vi "method parameters.Facade.vi"(0 "Data In":T5, 2 "Display State In":T3, 3 "Container State":T4) -> (6 "Data Out":T5, 7 "Display State Out":T3, 8 "Action":T2)   [LabVIEW 2014, in "method parameters.xctl"]
uses:
  method parameters.xctl
  method parameters.Data.ctl
  <vilib>/_xctls/Container State.ctl
  method parameters.State.ctl
  <vilib>/_xctls/Action.ctl
  <vilib>/_xctls/XControlSupport.lvlib
  CSlibraries/UtilityLib/UtilityLib.lvlib
  _common/PTUtils/PTUtils.lvlib
  CSCore/CSSystem/CoreLib/CoreLib.lvlib
panel:
  in  "Scrollbar":i32(c297)
  out "Indicator":T1
  in  "Control":T1
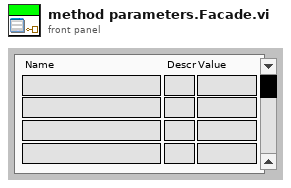
[diagram p1: front panel]
types:
  T1 = cluster{"Name 1":string, "Descr 1":string, "Value 1":string, "Name 2":string, "Descr 2":string, "Value 2":string, "Name 3":string, "Descr 3":string, "Value 3":string, "Name 4":string, "Descr 4":string, "Value 4":string}
  T2 = typedef "XControlSupport.lvlib/Action.ctl" = cluster{"Data Changed?":bool, "State Changed?":bool, "Action Name":string}
  T3 = typedef "method parameters.xctl/method parameters.State.ctl" = cluster{"index":i32}
  T4 = typedef "XControlSupport.lvlib/Container State.ctl" = cluster{"Indicator?":bool, "Run Mode?":bool, " Refnum":refnum<vi>}
  T5 = typedef "method parameters.xctl/method parameters.Data.ctl" = cluster{"Name":string, "Descr":string, "Value":string}[]
  T6 = enum8{"Enabled", "Disabled", "Disabled and Grayed Out"}
  T7 = cluster{"Name":string, "Descr":string, "Value":string}
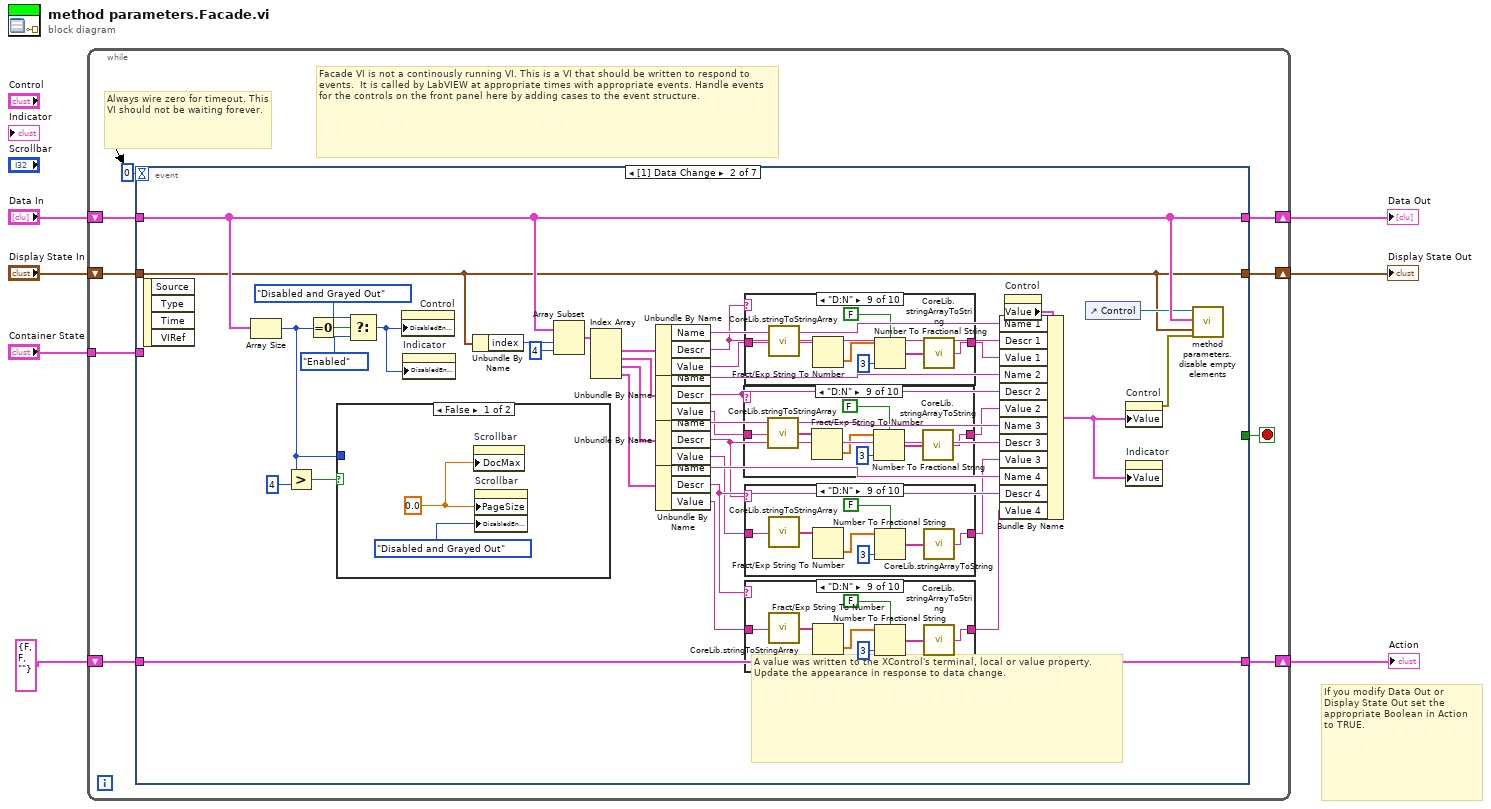
[diagram p0: block diagram]
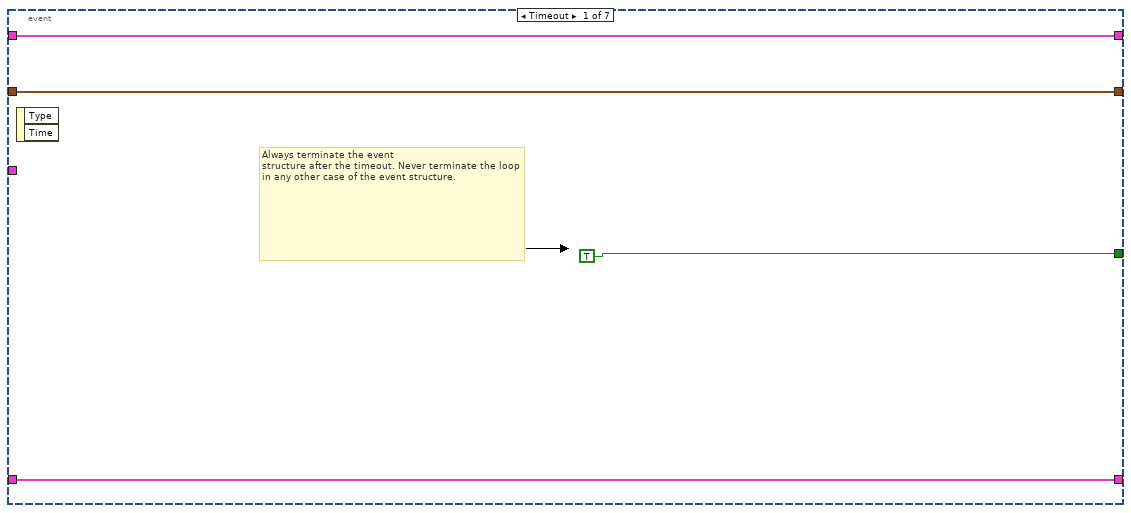
[diagram p2: hidden frame]
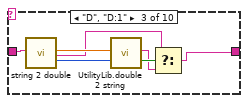
[diagram p5: hidden frame]
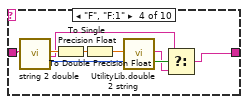
[diagram p6: hidden frame]
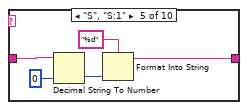
[diagram p7: hidden frame]
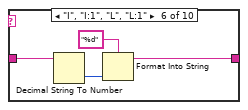
[diagram p8: hidden frame]
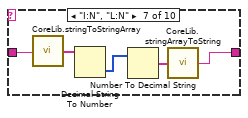
[diagram p9: hidden frame]
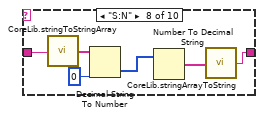
[diagram p10: hidden frame]
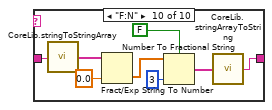
[diagram p11: hidden frame]
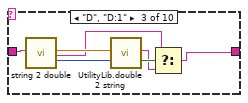
[diagram p14: hidden frame]
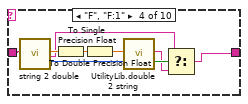
[diagram p15: hidden frame]
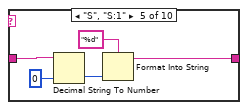
[diagram p16: hidden frame]
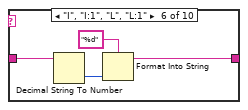
[diagram p17: hidden frame]
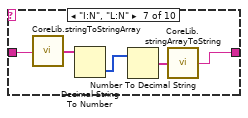
[diagram p18: hidden frame]
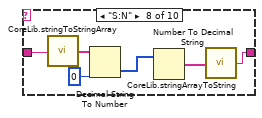
[diagram p19: hidden frame]
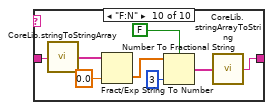
[diagram p20: hidden frame]
diagram:
  # "If you modify Data Out or\nDisplay State Out set the\nappropriate Boolean in Action\nto TRUE."
  n1 = while {
    shift-right: [w15] -> w4
    shift-left: "Display State In" -> [w16]
    tunnel: "Container State" -> [w12]
    shift-right: [w10] -> w7
    shift-left: "Data In" -> [w11]
    shift-right: [w8] -> w2
    shift-left: T2 {"Data Changed?"=FALSE, "State Changed?"=FALSE, "Action Name"=""} ("Action") -> [w9]
    stop <- w14 stop-if-true
    # "Facade VI is not a continously running VI. This is a VI that should be written to respond to events.  It is called by LabVIEW at appropriate times with appropriate events. Handle events for the controls on the front panel here by adding cases to the event structure."
    # "Always wire zero for timeout. This\nVI should not be waiting forever."
    n2 = event shown="[1] Data Change" {
      selector: _ -> [_ _ _ _ _ _ _]
      dyn-events: _ -> [_ _ _ _ _ _ _]
      timeout: 0 -> [_ _ _ _ _ _ _]
      tunnel: w16 -> [w18 w34 w280 w323 w327 w334 w384]
      tunnel: [w18 w34 w280 w323 w327 w329 w384] -> w15
      tunnel: [TRUE _ _ _ _ _ _] -> w14
      tunnel: w12 -> [_ _ _ w324 w328 _ _]
      tunnel: w11 -> [w17 w36 w279 w322 w326 w330 w383]
      tunnel: [w17 w36 w279 w322 w326 w330 w382] -> w10
      tunnel: [w19 w57 w309 w321 w325 w335 w395] -> w8
      tunnel: w9 -> [w19 w57 w309 w321 w325 w336 w396]
      event Timeout {
        # "Always terminate the event\nstructure after the timeout. Never terminate the loop in any other case of the event structure."
        n3 = event-data() -> ()  [unwired: 1 in, 2 out]
      }
      event Data Change {
        # "A value was written to the XControl's terminal, local or value property.\nUpdate the appearance in response to data change."
        n4 = event-data() -> ()  [unwired: 1 in, 4 out]
        n5 = Array Size(array=w36) -> (size(s)=w50:i32)
        n6 = Greater?(x=w50, y=4) -> (0:w56:bool)
        n7 = Equal To 0?(x=w50) -> (x = 0?=w53:bool)
        n8 = case shown="False" w56 {
          tunnel: w50 -> [_ w274]
          frame False {
            w270 = 0.0
            n9 = property on="Scrollbar" class="Scroll (strict)"("DocMax"=w270) -> ()  [unwired: 2 in, 2 out]
            n10 = property on="Scrollbar" class="Scroll (strict)"("PageSize"=w270, "DisabledEnum"=T6."Disabled and Grayed Out" ("Disabled")) -> ()  [unwired: 2 in, 2 out]
          }
          frame True {
            n11 = Subtract(x=w274, y=3) -> (x-y=w276:i32)
            n12 = To Double Precision Float(number=w274) -> (double precision float=w273:dbl)
            n13 = To Double Precision Float(number=w276) -> (double precision float=w275:dbl)
            n14 = property on="Scrollbar" class="Scroll (strict)"("DocMax"=w275, "DisabledEnum"=T6."Enabled" ("Disabled")) -> ()  [unwired: 2 in, 2 out]
            n15 = Divide(x=w275, y=w273) -> (x/y=w277:dbl)
            n16 = property on="Scrollbar" class="Scroll (strict)"("PageSize"=w277) -> ()  [unwired: 2 in, 2 out]
          }
        }
        n17 = Select(t=T6."Disabled and Grayed Out" ("Disabled"), s=w53, f=T6."Enabled" ("Disabled")) -> (s? t:f=w54:T6)
        n18 = property on="Control" class="Clust (strict)"("DisabledEnum"=w54) -> ()  [unwired: 2 in, 2 out]
        n19 = property on="Indicator" class="Clust (strict)"("DisabledEnum"=w54) -> ()  [unwired: 2 in, 2 out]
        n20 = Unbundle By Name(w34) -> ("index"=w48:i32)
        n21 = Array Subset(array=w36, index=w48, length=4) -> (w43:T5)
        n22 = Index Array(array=w43) -> (element #1=w42:T7, element #2=w41:T7, element #3=w40:T7, element #4=w39:T7)  [unwired: 4 in]
        n23 = Unbundle By Name(w42) -> ("Name"=w44:string, "Descr"=w32:string, "Value"=w31:string)
        n24 = Unbundle By Name(w41) -> ("Name"=w45:string, "Descr"=w21:string, "Value"=w23:string)
        n25 = Unbundle By Name(w40) -> ("Name"=w46:string, "Descr"=w25:string, "Value"=w26:string)
        n26 = Unbundle By Name(w39) -> ("Name"=w47:string, "Descr"=w27:string, "Value"=w29:string)
        n27 = case shown="\"D:N\"" w21 {
          tunnel: [w164 w165 w166 w173 w183 w188 w192 w200 w208 w216] -> w22
          tunnel: w23 -> [w164 w165 w170 w177 w182 w187 w191 w196 w203 w210]
          frame Default {
          }
          frame "C", "C:1", "C:N" {
          }
          frame "D", "D:1" {
            n28 = call "string 2 double.vi"("string"=w170) -> ("number"=w171:dbl, "scanned string"=w167:string, "length"=w172:u8)  [unwired: 15 in, 1 out]
            n29 = call "UtilityLib.double 2 string.vi"("Numeric"=w171, "length"=w172) -> ("String"=w168:string, "loss free"=w169:bool)  [unwired: 16 in]
            n30 = Select(t=w167, s=w169, f=w168) -> (s? t:f=w166:string)
          }
          frame "F", "F:1" {
            n31 = call "string 2 double.vi"("string"=w177) -> ("number"=w179:dbl, "scanned string"=w174:string, "length"=w181:u8)  [unwired: 15 in, 1 out]
            n32 = To Single Precision Float(number=w179) -> (single precision float=w180:sgl)
            n33 = To Double Precision Float(number=w180) -> (double precision float=w178:dbl)
            n34 = call "UtilityLib.double 2 string.vi"("Numeric"=w178, "length"=w181) -> ("String"=w175:string, "loss free"=w176:bool)  [unwired: 16 in]
            n35 = Select(t=w174, s=w176, f=w175) -> (s? t:f=w173:string)
          }
          frame "S", "S:1" {
            n36 = Decimal String To Number(string=w182, default (0L)=i16 0) -> (number=w185:i16)  [unwired: 1 in, 1 out]
            n37 = Format Into String(format string="%d", w185) -> (resulting string=w183:string)  [unwired: 2 in, 1 out]
          }
          frame "I", "I:1", "L", "L:1" {
            n38 = Decimal String To Number(string=w187) -> (number=w190:i32)  [unwired: 2 in, 1 out]
            n39 = Format Into String(format string="%d", w190) -> (resulting string=w188:string)  [unwired: 2 in, 1 out]
          }
          frame "I:N", "L:N" {
            n40 = call "CoreLib.stringToStringArray.vi"("String"=w191) -> ("Array"=w195:string[])
            n41 = Decimal String To Number(string=w195) -> (number=w194:i32[])  [unwired: 2 in, 1 out]
            n42 = Number To Decimal String(number=w194) -> (decimal integer string=w193:string[])  [unwired: 1 in]
            n43 = call "CoreLib.stringArrayToString.vi"("Array"=w193) -> ("String"=w192:string)
          }
          frame "S:N" {
            n44 = call "CoreLib.stringToStringArray.vi"("String"=w196) -> ("Array"=w201:string[])
            n45 = Decimal String To Number(string=w201, default (0L)=i16 0 ("default (0 I32)")) -> (number=w198:i16[])  [unwired: 1 in, 1 out]
            n46 = Number To Decimal String(number=w198) -> (decimal integer string=w197:string[])  [unwired: 1 in]
            n47 = call "CoreLib.stringArrayToString.vi"("Array"=w197) -> ("String"=w200:string)
          }
          frame "D:N" {
            n48 = call "CoreLib.stringToStringArray.vi"("String"=w203) -> ("Array"=w206:string[])
            n49 = Fract/Exp String To Number(string=w206) -> (number=w205:dbl[])  [unwired: 3 in, 1 out]
            n50 = Number To Fractional String(use system decimal point (T)=FALSE, number=w205, precision (6)=i16 3) -> (F-format string=w204:string[])  [unwired: 1 in]
            n51 = call "CoreLib.stringArrayToString.vi"("Array"=w204) -> ("String"=w208:string)
          }
          frame "F:N" {
            n52 = call "CoreLib.stringToStringArray.vi"("String"=w210) -> ("Array"=w214:string[])
            n53 = Fract/Exp String To Number(string=w214, default (0 dbl)=sgl 0.0 ("default (0 DBL)")) -> (number=w211:sgl[])  [unwired: 2 in, 1 out]
            n54 = Number To Fractional String(use system decimal point (T)=FALSE, number=w211, precision (6)=i16 3) -> (F-format string=w213:string[])  [unwired: 1 in]
            n55 = call "CoreLib.stringArrayToString.vi"("Array"=w213) -> ("String"=w216:string)
          }
        }
        n56 = case shown="\"D:N\"" w32 {
          tunnel: [w217 w218 w219 w226 w236 w241 w245 w253 w261 w269] -> w30
          tunnel: w31 -> [w217 w218 w223 w230 w235 w240 w244 w249 w256 w263]
          frame Default {
          }
          frame "C", "C:1", "C:N" {
          }
          frame "D", "D:1" {
            n57 = call "string 2 double.vi"("string"=w223) -> ("number"=w224:dbl, "scanned string"=w220:string, "length"=w225:u8)  [unwired: 15 in, 1 out]
            n58 = call "UtilityLib.double 2 string.vi"("Numeric"=w224, "length"=w225) -> ("String"=w221:string, "loss free"=w222:bool)  [unwired: 16 in]
            n59 = Select(t=w220, s=w222, f=w221) -> (s? t:f=w219:string)
          }
          frame "F", "F:1" {
            n60 = call "string 2 double.vi"("string"=w230) -> ("number"=w232:dbl, "scanned string"=w227:string, "length"=w234:u8)  [unwired: 15 in, 1 out]
            n61 = To Single Precision Float(number=w232) -> (single precision float=w233:sgl)
            n62 = To Double Precision Float(number=w233) -> (double precision float=w231:dbl)
            n63 = call "UtilityLib.double 2 string.vi"("Numeric"=w231, "length"=w234) -> ("String"=w228:string, "loss free"=w229:bool)  [unwired: 16 in]
            n64 = Select(t=w227, s=w229, f=w228) -> (s? t:f=w226:string)
          }
          frame "S", "S:1" {
            n65 = Decimal String To Number(string=w235, default (0L)=i16 0) -> (number=w238:i16)  [unwired: 1 in, 1 out]
            n66 = Format Into String(format string="%d", w238) -> (resulting string=w236:string)  [unwired: 2 in, 1 out]
          }
          frame "I", "I:1", "L", "L:1" {
            n67 = Decimal String To Number(string=w240) -> (number=w243:i32)  [unwired: 2 in, 1 out]
            n68 = Format Into String(format string="%d", w243) -> (resulting string=w241:string)  [unwired: 2 in, 1 out]
          }
          frame "I:N", "L:N" {
            n69 = call "CoreLib.stringToStringArray.vi"("String"=w244) -> ("Array"=w248:string[])
            n70 = Decimal String To Number(string=w248) -> (number=w247:i32[])  [unwired: 2 in, 1 out]
            n71 = Number To Decimal String(number=w247) -> (decimal integer string=w246:string[])  [unwired: 1 in]
            n72 = call "CoreLib.stringArrayToString.vi"("Array"=w246) -> ("String"=w245:string)
          }
          frame "S:N" {
            n73 = call "CoreLib.stringToStringArray.vi"("String"=w249) -> ("Array"=w254:string[])
            n74 = Decimal String To Number(string=w254, default (0L)=i16 0 ("default (0 I32)")) -> (number=w251:i16[])  [unwired: 1 in, 1 out]
            n75 = Number To Decimal String(number=w251) -> (decimal integer string=w250:string[])  [unwired: 1 in]
            n76 = call "CoreLib.stringArrayToString.vi"("Array"=w250) -> ("String"=w253:string)
          }
          frame "D:N" {
            n77 = call "CoreLib.stringToStringArray.vi"("String"=w256) -> ("Array"=w259:string[])
            n78 = Fract/Exp String To Number(string=w259) -> (number=w258:dbl[])  [unwired: 3 in, 1 out]
            n79 = Number To Fractional String(use system decimal point (T)=FALSE, number=w258, precision (6)=i16 3) -> (F-format string=w257:string[])  [unwired: 1 in]
            n80 = call "CoreLib.stringArrayToString.vi"("Array"=w257) -> ("String"=w261:string)
          }
          frame "F:N" {
            n81 = call "CoreLib.stringToStringArray.vi"("String"=w263) -> ("Array"=w267:string[])
            n82 = Fract/Exp String To Number(string=w267, default (0 dbl)=sgl 0.0 ("default (0 DBL)")) -> (number=w264:sgl[])  [unwired: 2 in, 1 out]
            n83 = Number To Fractional String(use system decimal point (T)=FALSE, number=w264, precision (6)=i16 3) -> (F-format string=w266:string[])  [unwired: 1 in]
            n84 = call "CoreLib.stringArrayToString.vi"("Array"=w266) -> ("String"=w269:string)
          }
        }
        n85 = case shown="\"D:N\"" w25 {
          tunnel: [w111 w112 w113 w120 w130 w135 w139 w147 w155 w163] -> w24
          tunnel: w26 -> [w111 w112 w117 w124 w129 w134 w138 w143 w150 w157]
          frame Default {
          }
          frame "C", "C:1", "C:N" {
          }
          frame "D", "D:1" {
            n86 = call "string 2 double.vi"("string"=w117) -> ("number"=w118:dbl, "scanned string"=w114:string, "length"=w119:u8)  [unwired: 15 in, 1 out]
            n87 = call "UtilityLib.double 2 string.vi"("Numeric"=w118, "length"=w119) -> ("String"=w115:string, "loss free"=w116:bool)  [unwired: 16 in]
            n88 = Select(t=w114, s=w116, f=w115) -> (s? t:f=w113:string)
          }
          frame "F", "F:1" {
            n89 = call "string 2 double.vi"("string"=w124) -> ("number"=w126:dbl, "scanned string"=w121:string, "length"=w128:u8)  [unwired: 15 in, 1 out]
            n90 = To Single Precision Float(number=w126) -> (single precision float=w127:sgl)
            n91 = To Double Precision Float(number=w127) -> (double precision float=w125:dbl)
            n92 = call "UtilityLib.double 2 string.vi"("Numeric"=w125, "length"=w128) -> ("String"=w122:string, "loss free"=w123:bool)  [unwired: 16 in]
            n93 = Select(t=w121, s=w123, f=w122) -> (s? t:f=w120:string)
          }
          frame "S", "S:1" {
            n94 = Decimal String To Number(string=w129, default (0L)=i16 0) -> (number=w132:i16)  [unwired: 1 in, 1 out]
            n95 = Format Into String(format string="%d", w132) -> (resulting string=w130:string)  [unwired: 2 in, 1 out]
          }
          frame "I", "I:1", "L", "L:1" {
            n96 = Decimal String To Number(string=w134) -> (number=w137:i32)  [unwired: 2 in, 1 out]
            n97 = Format Into String(format string="%d", w137) -> (resulting string=w135:string)  [unwired: 2 in, 1 out]
          }
          frame "I:N", "L:N" {
            n98 = call "CoreLib.stringToStringArray.vi"("String"=w138) -> ("Array"=w142:string[])
            n99 = Decimal String To Number(string=w142) -> (number=w141:i32[])  [unwired: 2 in, 1 out]
            n100 = Number To Decimal String(number=w141) -> (decimal integer string=w140:string[])  [unwired: 1 in]
            n101 = call "CoreLib.stringArrayToString.vi"("Array"=w140) -> ("String"=w139:string)
          }
          frame "S:N" {
            n102 = call "CoreLib.stringToStringArray.vi"("String"=w143) -> ("Array"=w148:string[])
            n103 = Decimal String To Number(string=w148, default (0L)=i16 0 ("default (0 I32)")) -> (number=w145:i16[])  [unwired: 1 in, 1 out]
            n104 = Number To Decimal String(number=w145) -> (decimal integer string=w144:string[])  [unwired: 1 in]
            n105 = call "CoreLib.stringArrayToString.vi"("Array"=w144) -> ("String"=w147:string)
          }
          frame "D:N" {
            n106 = call "CoreLib.stringToStringArray.vi"("String"=w150) -> ("Array"=w153:string[])
            n107 = Fract/Exp String To Number(string=w153) -> (number=w152:dbl[])  [unwired: 3 in, 1 out]
            n108 = Number To Fractional String(use system decimal point (T)=FALSE, number=w152, precision (6)=i16 3) -> (F-format string=w151:string[])  [unwired: 1 in]
            n109 = call "CoreLib.stringArrayToString.vi"("Array"=w151) -> ("String"=w155:string)
          }
          frame "F:N" {
            n110 = call "CoreLib.stringToStringArray.vi"("String"=w157) -> ("Array"=w161:string[])
            n111 = Fract/Exp String To Number(string=w161, default (0 dbl)=sgl 0.0 ("default (0 DBL)")) -> (number=w158:sgl[])  [unwired: 2 in, 1 out]
            n112 = Number To Fractional String(use system decimal point (T)=FALSE, number=w158, precision (6)=i16 3) -> (F-format string=w160:string[])  [unwired: 1 in]
            n113 = call "CoreLib.stringArrayToString.vi"("Array"=w160) -> ("String"=w163:string)
          }
        }
        n114 = case shown="\"D:N\"" w27 {
          tunnel: [w58 w59 w60 w67 w77 w82 w86 w94 w102 w110] -> w28
          tunnel: w29 -> [w58 w59 w64 w71 w76 w81 w85 w90 w97 w104]
          frame Default {
          }
          frame "C", "C:1", "C:N" {
          }
          frame "D", "D:1" {
            n115 = call "string 2 double.vi"("string"=w64) -> ("number"=w65:dbl, "scanned string"=w61:string, "length"=w66:u8)  [unwired: 15 in, 1 out]
            n116 = call "UtilityLib.double 2 string.vi"("Numeric"=w65, "length"=w66) -> ("String"=w62:string, "loss free"=w63:bool)  [unwired: 16 in]
            n117 = Select(t=w61, s=w63, f=w62) -> (s? t:f=w60:string)
          }
          frame "F", "F:1" {
            n118 = call "string 2 double.vi"("string"=w71) -> ("number"=w73:dbl, "scanned string"=w68:string, "length"=w75:u8)  [unwired: 15 in, 1 out]
            n119 = To Single Precision Float(number=w73) -> (single precision float=w74:sgl)
            n120 = To Double Precision Float(number=w74) -> (double precision float=w72:dbl)
            n121 = call "UtilityLib.double 2 string.vi"("Numeric"=w72, "length"=w75) -> ("String"=w69:string, "loss free"=w70:bool)  [unwired: 16 in]
            n122 = Select(t=w68, s=w70, f=w69) -> (s? t:f=w67:string)
          }
          frame "S", "S:1" {
            n123 = Decimal String To Number(string=w76, default (0L)=i16 0) -> (number=w79:i16)  [unwired: 1 in, 1 out]
            n124 = Format Into String(format string="%d", w79) -> (resulting string=w77:string)  [unwired: 2 in, 1 out]
          }
          frame "I", "I:1", "L", "L:1" {
            n125 = Decimal String To Number(string=w81) -> (number=w84:i32)  [unwired: 2 in, 1 out]
            n126 = Format Into String(format string="%d", w84) -> (resulting string=w82:string)  [unwired: 2 in, 1 out]
          }
          frame "I:N", "L:N" {
            n127 = call "CoreLib.stringToStringArray.vi"("String"=w85) -> ("Array"=w89:string[])
            n128 = Decimal String To Number(string=w89) -> (number=w88:i32[])  [unwired: 2 in, 1 out]
            n129 = Number To Decimal String(number=w88) -> (decimal integer string=w87:string[])  [unwired: 1 in]
            n130 = call "CoreLib.stringArrayToString.vi"("Array"=w87) -> ("String"=w86:string)
          }
          frame "S:N" {
            n131 = call "CoreLib.stringToStringArray.vi"("String"=w90) -> ("Array"=w95:string[])
            n132 = Decimal String To Number(string=w95, default (0L)=i16 0 ("default (0 I32)")) -> (number=w92:i16[])  [unwired: 1 in, 1 out]
            n133 = Number To Decimal String(number=w92) -> (decimal integer string=w91:string[])  [unwired: 1 in]
            n134 = call "CoreLib.stringArrayToString.vi"("Array"=w91) -> ("String"=w94:string)
          }
          frame "D:N" {
            n135 = call "CoreLib.stringToStringArray.vi"("String"=w97) -> ("Array"=w100:string[])
            n136 = Fract/Exp String To Number(string=w100) -> (number=w99:dbl[])  [unwired: 3 in, 1 out]
            n137 = Number To Fractional String(use system decimal point (T)=FALSE, number=w99, precision (6)=i16 3) -> (F-format string=w98:string[])  [unwired: 1 in]
            n138 = call "CoreLib.stringArrayToString.vi"("Array"=w98) -> ("String"=w102:string)
          }
          frame "F:N" {
            n139 = call "CoreLib.stringToStringArray.vi"("String"=w104) -> ("Array"=w108:string[])
            n140 = Fract/Exp String To Number(string=w108, default (0 dbl)=sgl 0.0 ("default (0 DBL)")) -> (number=w105:sgl[])  [unwired: 2 in, 1 out]
            n141 = Number To Fractional String(use system decimal point (T)=FALSE, number=w105, precision (6)=i16 3) -> (F-format string=w107:string[])  [unwired: 1 in]
            n142 = call "CoreLib.stringArrayToString.vi"("Array"=w107) -> ("String"=w110:string)
          }
        }
        n143 = property on="Control" class="Clust (strict)"() -> ("Value"=w38:T1)  [unwired: 2 in, 2 out]
        n144 = Bundle By Name(cluster=w38, "Name 1"=w44, "Descr 1"=w32, "Value 1"=w30, "Name 2"=w45, "Descr 2"=w21, "Value 2"=w22, "Name 3"=w46, "Descr 3"=w25, "Value 3"=w24, "Name 4"=w47, "Descr 4"=w27, "Value 4"=w28) -> (w37:T1)
        n145 = control-ref of="Control"() -> (w35:refnum<vi>)
        n146 = property on="Control" class="Clust (strict)"("Value"=w37) -> (error out=w33:errorcluster)  [unwired: 2 in, 1 out]
        n147 = property on="Indicator" class="Clust (strict)"("Value"=w37) -> ()  [unwired: 2 in, 2 out]
        n148 = call "method parameters.disable empty elements.vi"("control ref"=w35, "Data In"=w36, "State"=w34, "error in (no error)"=w33) -> ()  [unwired: 15 in, 1 out]
      }
      event Display State Change {
        # "Display State changed as a result of dropping a new instance of this XControl, copying, undoing an operation or executing a custom property or method on this XControl. Update the appearance accordingly."
        n149 = event-data() -> ()  [unwired: 1 in, 4 out]
        n150 = Array Size(array=w279) -> (size(s)=w302:i32)
        n151 = Greater?(x=w302, y=4) -> (0:w308:bool)
        n152 = case shown="False" w308 {
          tunnel: w302 -> [_ w314]
          frame False {
            w310 = 0.0
            n153 = property on="Scrollbar" class="Scroll (strict)"("DocMax"=w310) -> ()  [unwired: 2 in, 2 out]
            n154 = property on="Scrollbar" class="Scroll (strict)"("PageSize"=w310, "DisabledEnum"=T6."Disabled and Grayed Out" ("Disabled")) -> ()  [unwired: 2 in, 2 out]
          }
          frame True {
            n155 = Subtract(x=w314, y=3) -> (x-y=w316:i32)
            n156 = To Double Precision Float(number=w314) -> (double precision float=w313:dbl)
            n157 = To Double Precision Float(number=w316) -> (double precision float=w315:dbl)
            n158 = property on="Scrollbar" class="Scroll (strict)"("DocMax"=w315, "DisabledEnum"=T6."Enabled" ("Disabled")) -> ()  [unwired: 2 in, 2 out]
            n159 = Divide(x=w315, y=w313) -> (x/y=w317:dbl)
            n160 = property on="Scrollbar" class="Scroll (strict)"("PageSize"=w317) -> ()  [unwired: 2 in, 2 out]
          }
        }
        n161 = Equal To 0?(x=w302) -> (x = 0?=w305:bool)
        n162 = Select(t=T6."Disabled and Grayed Out" ("Disabled"), s=w305, f=T6."Enabled" ("Disabled")) -> (s? t:f=w306:T6)
        n163 = property on="Control" class="Clust (strict)"("DisabledEnum"=w306) -> ()  [unwired: 2 in, 2 out]
        n164 = property on="Indicator" class="Clust (strict)"("DisabledEnum"=w306) -> ()  [unwired: 2 in, 2 out]
        n165 = Unbundle By Name(w280) -> ("index"=w300:i32)
        n166 = Array Subset(array=w279, index=w300, length=4) -> (w287:T5)
        n167 = Index Array(array=w287) -> (element #1=w286:T7, element #2=w285:T7, element #3=w284:T7, element #4=w283:T7)  [unwired: 4 in]
        n168 = Unbundle By Name(w286) -> ("Name"=w288:string, "Descr"=w289:string, "Value"=w290:string)
        n169 = Unbundle By Name(w285) -> ("Name"=w291:string, "Descr"=w292:string, "Value"=w293:string)
        n170 = Unbundle By Name(w284) -> ("Name"=w294:string, "Descr"=w295:string, "Value"=w296:string)
        n171 = Unbundle By Name(w283) -> ("Name"=w297:string, "Descr"=w298:string, "Value"=w299:string)
        n172 = property on="Control" class="Clust (strict)"() -> ("Value"=w282:T1)  [unwired: 2 in, 2 out]
        n173 = Bundle By Name(cluster=w282, "Name 1"=w288, "Descr 1"=w289, "Value 1"=w290, "Name 2"=w291, "Descr 2"=w292, "Value 2"=w293, "Name 3"=w294, "Descr 3"=w295, "Value 3"=w296, "Name 4"=w297, "Descr 4"=w298, "Value 4"=w299) -> (w281:T1)
        n174 = property on="Control" class="Clust (strict)"("Value"=w281) -> ()  [unwired: 2 in, 2 out]
        n175 = property on="Indicator" class="Clust (strict)"("Value"=w281) -> ()  [unwired: 2 in, 2 out]
      }
      event Direction Change {
        # "The direction of the XControl changed from a control to an indicator or vice versa. Update the appearance accordingly."
        n176 = event-data() -> ()  [unwired: 1 in, 4 out]
        n177 = Unbundle By Name(w324) -> ("Indicator?"=w320:bool)
        n178 = Not(x=w320) -> (.not. x?=w319:bool)
        n179 = property on="Indicator" class="Clust (strict)"("Visible"=w320) -> ()  [unwired: 2 in, 2 out]
        n180 = property on="Control" class="Clust (strict)"("Visible"=w319) -> ()  [unwired: 2 in, 2 out]
      }
      event Exec State Change {
        # "The VI owning the XControl changed from Edit Mode  to Run Mode or vice versa.\nUpdate the appearance accordingly."
        # "Handle Edit Mode & Run Mode\ncase differently"
        n181 = event-data() -> ()  [unwired: 1 in, 4 out]
        n182 = Unbundle By Name(w328) -> ()  [unwired: 1 out]
      }
      event "Scrollbar": Value Change {
        n183 = event-data() -> ("OldVal"=w333:i32, "NewVal"=w332:i32)  [unwired: 1 in, 4 out]
        n184 = Unbundle By Name(w334) -> ("index"=w338:i32)
        n185 = Array Size(array=w330) -> (size(s)=w340:i32)
        n186 = Add(x=w338, y=4) -> (x+y=w341:i32)
        n187 = Equal To 0?(x=w333) -> (x = 0?=w345:bool)
        n188 = Equal?(x=w340, y=w341) -> (x = y?=w342:bool)
        n189 = Less?(x=w333, y=w332) -> (x < y?=w344:bool)
        n190 = And(x=w342, y=w344) -> (x .and. y?=w347:bool)
        n191 = Not(x=w344) -> (.not. x?=w343:bool)
        n192 = And(x=w343, y=w345) -> (x .and. y?=w346:bool)
        n193 = Or(x=w347, y=w346) -> (x .or. y?=w337:bool)
        n194 = case shown="False" w337 {
          tunnel: w336 -> [w373 w377]
          tunnel: [w372 w377] -> w335
          tunnel: [w370 w376] -> w329
          tunnel: w334 -> [w371 w376]
          tunnel: w333 -> [_ w375]
          tunnel: w332 -> [w367 _]
          tunnel: w330 -> [w368 _]
          frame False {
            n195 = Bundle By Name(cluster=w371, "index"=w367) -> (w370:T3)
            n196 = Array Subset(array=w368, index=w367, length=4) -> (w354:T5)
            n197 = Index Array(array=w354) -> (element #1=w353:T7, element #2=w352:T7, element #3=w351:T7, element #4=w350:T7)  [unwired: 4 in]
            n198 = Unbundle By Name(w353) -> ("Name"=w355:string, "Descr"=w356:string, "Value"=w357:string)
            n199 = Unbundle By Name(w352) -> ("Name"=w358:string, "Descr"=w359:string, "Value"=w360:string)
            n200 = Unbundle By Name(w351) -> ("Name"=w361:string, "Descr"=w362:string, "Value"=w363:string)
            n201 = Unbundle By Name(w350) -> ("Name"=w364:string, "Descr"=w365:string, "Value"=w366:string)
            n202 = Bundle By Name(cluster=w373, "State Changed?"=TRUE) -> (w372:T2)
            n203 = property on="Control" class="Clust (strict)"() -> ("Value"=w349:T1)  [unwired: 2 in, 2 out]
            n204 = Bundle By Name(cluster=w349, "Name 1"=w355, "Descr 1"=w356, "Value 1"=w357, "Name 2"=w358, "Descr 2"=w359, "Value 2"=w360, "Name 3"=w361, "Descr 3"=w362, "Value 3"=w363, "Name 4"=w364, "Descr 4"=w365, "Value 4"=w366) -> (w348:T1)
            n205 = property on="Control" class="Clust (strict)"("Value"=w348) -> ()  [unwired: 2 in, 2 out]
            n206 = property on="Indicator" class="Clust (strict)"("Value"=w348) -> ()  [unwired: 2 in, 2 out]
          }
          frame True {
            n207 = property on="Scrollbar" class="Scroll (strict)"("Value"=w375) -> ()  [unwired: 2 in, 2 out]
          }
        }
        n208 = control-ref of="Control"() -> (w331:refnum<vi>)
        n209 = call "method parameters.disable empty elements.vi"("control ref"=w331, "Data In"=w330, "State"=w329) -> ()  [unwired: 16 in, 1 out]
      }
      event "Control.Value 1", "Control.Value 2", "Control.Value 3", "Control.Value 4": Value Change {
        n210 = event-data() -> ("CtlRef"=w379:refnum<vi>, "NewVal"=w378:string, "OldVal"=w385:string)  [unwired: 1 in, 3 out]
        n211 = property class="Str"(reference=w379) -> ("Label.Text"=w386:string)  [unwired: 1 in, 2 out]
        n212 = Unbundle By Name(w384) -> ("index"=w388:i32)
        n213 = Scan From String(format string="%s %d", input string=w386) -> (output 2=w391:i32)  [unwired: 5 in, 3 out]
        n214 = Add(x=w388, y=w391) -> (x+y=w389:i32)
        n215 = Decrement(x=w389) -> (x-1=w394:i32)
        n216 = Index Array(array=w383, index=w394) -> (element=w393:T7)
        n217 = Unbundle By Name(w393) -> ("Descr"=w390:string)
        n218 = case shown="\"C\", \"C:1\", \"C:N\"" w390 {
          tunnel: w383 -> [w412 w417 w430 w450 w460 w471 w484 w495 w507 w520]
          tunnel: [w412 w418 w429 w449 w461 w470 w483 w494 w506 w519] -> w382
          tunnel: w378 -> [_ w413 w422 w443 w466 w475 w480 w491 w503 w516]
          tunnel: [w411 w413 w419 w437 w458 w468 w476 w489 w502 w515] -> w392
          tunnel: w393 -> [_ w415 w421 w442 w459 w469 w482 w493 w505 w518]
          tunnel: w394 -> [_ w416 w428 w448 w457 w467 w481 w492 w504 w517]
          tunnel: w385 -> [w411 _ _ _ _ _ _ _ _ _]
          frame Default {
          }
          frame "C", "C:1", "C:N" {
            n219 = Bundle By Name(cluster=w415, "Value"=w413) -> (w414:T7)
            n220 = Replace Array Subset(array=w417, new element=w414, index=w416) -> (w418:T5)
          }
          frame "D", "D:1" {
            n221 = call "string 2 double.vi"("string"=w422) -> ("number"=w423:dbl, "scanned string"=w426:string, "length"=w424:u8)  [unwired: 15 in, 1 out]
            n222 = call "UtilityLib.double 2 string.vi"("Numeric"=w423, "length"=w424) -> ("String"=w427:string, "loss free"=w425:bool)  [unwired: 16 in]
            n223 = case shown="False" w425 {
              tunnel: [w433 w436] -> w420
              tunnel: w426 -> [w432 _]
              tunnel: [w432 w435] -> w419
              tunnel: w427 -> [_ w435]
              tunnel: w421 -> [w431 w434]
              frame True {
                n224 = Bundle By Name(cluster=w431, "Value"=w432) -> (w433:T7)
              }
              frame False {
                n225 = Bundle By Name(cluster=w434, "Value"=w435) -> (w436:T7)
              }
            }
            n226 = Replace Array Subset(array=w430, new element=w420, index=w428) -> (w429:T5)
          }
          frame "F", "F:1" {
            n227 = call "string 2 double.vi"("string"=w443) -> ("number"=w439:dbl, "scanned string"=w446:string, "length"=w444:u8)  [unwired: 15 in, 1 out]
            n228 = To Single Precision Float(number=w439) -> (single precision float=w440:sgl)
            n229 = To Double Precision Float(number=w440) -> (double precision float=w438:dbl)
            n230 = call "UtilityLib.double 2 string.vi"("Numeric"=w438, "length"=w444) -> ("String"=w447:string, "loss free"=w445:bool)  [unwired: 16 in]
            n231 = case shown="True" w445 {
              tunnel: [w453 w456] -> w441
              tunnel: w446 -> [w452 _]
              tunnel: [w452 w455] -> w437
              tunnel: w447 -> [_ w455]
              tunnel: w442 -> [w451 w454]
              frame True {
                n232 = Bundle By Name(cluster=w451, "Value"=w452) -> (w453:T7)
              }
              frame False {
                n233 = Bundle By Name(cluster=w454, "Value"=w455) -> (w456:T7)
              }
            }
            n234 = Replace Array Subset(array=w450, new element=w441, index=w448) -> (w449:T5)
          }
          frame "S", "S:1" {
            n235 = Decimal String To Number(string=w466, default (0L)=i16 0) -> (number=w464:i16)  [unwired: 1 in, 1 out]
            n236 = Format Into String(format string="%d", w464) -> (resulting string=w458:string)  [unwired: 2 in, 1 out]
            n237 = Bundle By Name(cluster=w459, "Value"=w458) -> (w462:T7)
            n238 = Replace Array Subset(array=w460, new element=w462, index=w457) -> (w461:T5)
          }
          frame "I", "I:1", "L", "L:1" {
            n239 = Decimal String To Number(string=w475) -> (number=w474:i32)  [unwired: 2 in, 1 out]
            n240 = Format Into String(format string="%d", w474) -> (resulting string=w468:string)  [unwired: 2 in, 1 out]
            n241 = Bundle By Name(cluster=w469, "Value"=w468) -> (w472:T7)
            n242 = Replace Array Subset(array=w471, new element=w472, index=w467) -> (w470:T5)
          }
          frame "I:N", "L:N" {
            n243 = call "CoreLib.stringToStringArray.vi"("String"=w480) -> ("Array"=w479:string[])
            n244 = Decimal String To Number(string=w479) -> (number=w478:i32[])  [unwired: 2 in, 1 out]
            n245 = Number To Decimal String(number=w478) -> (decimal integer string=w477:string[])  [unwired: 1 in]
            n246 = call "CoreLib.stringArrayToString.vi"("Array"=w477) -> ("String"=w476:string)
            n247 = Bundle By Name(cluster=w482, "Value"=w476) -> (w485:T7)
            n248 = Replace Array Subset(array=w484, new element=w485, index=w481) -> (w483:T5)
          }
          frame "S:N" {
            n249 = call "CoreLib.stringToStringArray.vi"("String"=w491) -> ("Array"=w490:string[])
            n250 = Decimal String To Number(string=w490, default (0L)=i16 0 ("default (0 I32)")) -> (number=w487:i16[])  [unwired: 1 in, 1 out]
            n251 = Number To Decimal String(number=w487) -> (decimal integer string=w486:string[])  [unwired: 1 in]
            n252 = call "CoreLib.stringArrayToString.vi"("Array"=w486) -> ("String"=w489:string)
            n253 = Bundle By Name(cluster=w493, "Value"=w489) -> (w496:T7)
            n254 = Replace Array Subset(array=w495, new element=w496, index=w492) -> (w494:T5)
          }
          frame "D:N" {
            n255 = call "CoreLib.stringToStringArray.vi"("String"=w503) -> ("Array"=w500:string[])
            n256 = Fract/Exp String To Number(string=w500) -> (number=w499:dbl[])  [unwired: 3 in, 1 out]
            n257 = Number To Fractional String(use system decimal point (T)=FALSE, number=w499, precision (6)=i16 3) -> (F-format string=w498:string[])  [unwired: 1 in]
            n258 = call "CoreLib.stringArrayToString.vi"("Array"=w498) -> ("String"=w502:string)
            n259 = Bundle By Name(cluster=w505, "Value"=w502) -> (w508:T7)
            n260 = Replace Array Subset(array=w507, new element=w508, index=w504) -> (w506:T5)
          }
          frame "F:N" {
            n261 = call "CoreLib.stringToStringArray.vi"("String"=w516) -> ("Array"=w513:string[])
            n262 = Fract/Exp String To Number(string=w513, default (0 dbl)=sgl 0.0 ("default (0 DBL)")) -> (number=w510:sgl[])  [unwired: 2 in, 1 out]
            n263 = Number To Fractional String(use system decimal point (T)=FALSE, number=w510, precision (6)=i16 3) -> (F-format string=w512:string[])  [unwired: 1 in]
            n264 = call "CoreLib.stringArrayToString.vi"("Array"=w512) -> ("String"=w515:string)
            n265 = Bundle By Name(cluster=w518, "Value"=w515) -> (w521:T7)
            n266 = Replace Array Subset(array=w520, new element=w521, index=w517) -> (w519:T5)
          }
        }
        n267 = Bundle By Name(cluster=w396, "Data Changed?"=TRUE) -> (w395:T2)
        n268 = property on="Control" class="Clust (strict)"() -> ("Value"=w381:T1)  [unwired: 2 in, 2 out]
        n269 = case shown="1" w391 {
          tunnel: w392 -> [_ w401 w404 w407 w410]
          tunnel: w381 -> [w398 w400 w403 w406 w409]
          tunnel: [w398 w399 w402 w405 w408] -> w380
          frame 0, Default {
          }
          frame 1 {
            n270 = Bundle By Name(cluster=w400, "Value 1"=w401) -> (w399:T1)
          }
          frame 2 {
            n271 = Bundle By Name(cluster=w403, "Value 2"=w404) -> (w402:T1)
          }
          frame 3 {
            n272 = Bundle By Name(cluster=w406, "Value 3"=w407) -> (w405:T1)
          }
          frame 4 {
            n273 = Bundle By Name(cluster=w409, "Value 4"=w410) -> (w408:T1)
          }
        }
        n274 = property on="Control" class="Clust (strict)"("Value"=w380) -> ()  [unwired: 2 in, 2 out]
        n275 = property on="Indicator" class="Clust (strict)"("Value"=w380) -> ()  [unwired: 2 in, 2 out]
      }
    }
  }
  "Display State Out" <- w4
  "Data Out" <- w7
  "Action" <- w2
